vi "INI_bk5492c.vi"(5 "MCListbox Ref":refnum<vi>, 9 "MListBox Row":u16=2 max=8, 11 "Device INI Config File Path":path=path "D:/LABVIEW/SEQUENSER SNA/Ver 07/INI/DeviceConfig.ini") -> (0 "error out":errorcluster, 3 "Serial_VISA":T1)   [LabVIEW 2018]
uses:
  Examples - 32bit/SEQUENCER/SEQUENSER v10/Sequencer v10/Ctl/Serial_VISA.ctl
  <vilib>/Utility/miscctls.llb/LVRowAndColumnTypeDef.ctl
  <vilib>/Utility/config.llb/Read Key (String).vi
  <vilib>/Utility/config.llb/NI_LVConfig.lvlib
  <instrlib>/BK Precision 5490C Series/BK Precision 5490C Series.lvlib
panel:
  out "Array DMM":string[](array[string])
  out "DMM Read Buffer":string
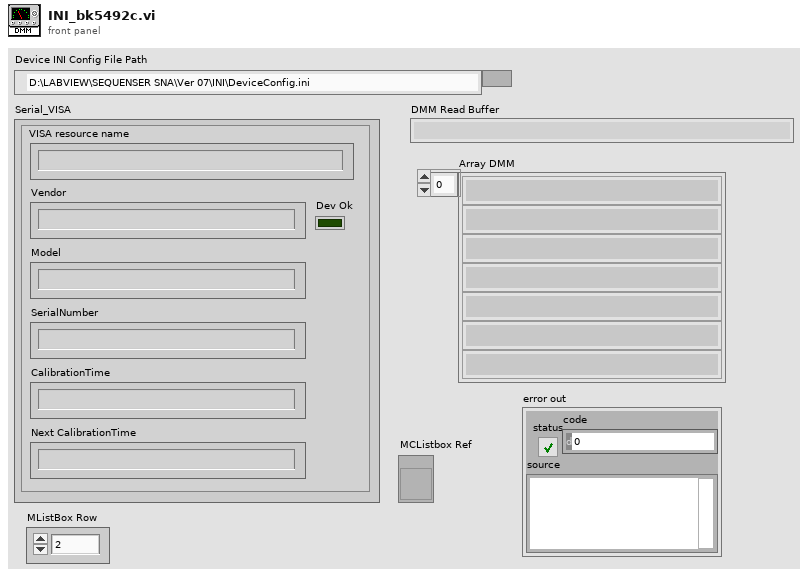
[diagram p1: front panel]
types:
  T1 = typedef "Serial_VISA.ctl" = cluster{"VISA resource name":string, "Vendor":string, "SerialNumber":string, "CalibrationTime":string, "Dev Ok":bool, "Model":string, "Next CalibrationTime":string}
  T2 = typedef "LVRowAndColumnTypeDef.ctl" = cluster{"Row":i32, "Column":i32}
  T3 = typedef "NI_LVConfig.lvlib/Config Data RefNum.ctl" = refnum<k1>
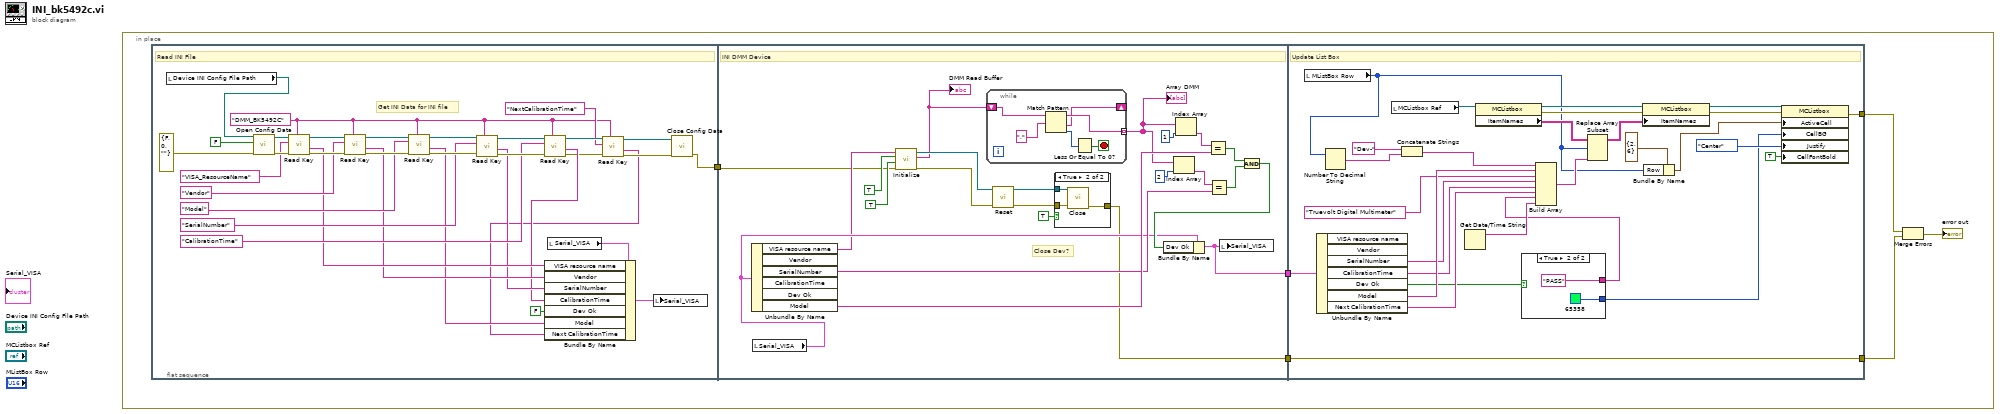
[diagram p0: block diagram]
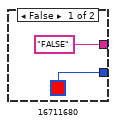
[diagram p3: hidden frame]
diagram:
  n1 = in-place {
    n2 = flat-sequence {
      tunnel: [w8] -> w6
      tunnel: w6 -> [w43]
      tunnel: [w49] -> w4
      tunnel: [w53] -> w1
      tunnel: [w81] -> w5
      tunnel: [w80] -> w3
      tunnel: w4 -> [w80]
      tunnel: w1 -> [w78]
      frame #0 {
        w13 = "DMM_BK5492C" ("section")
        # "Get INI Data for INI file"
        # "Read INI File"
        n3 = local read "Device INI Config File Path"() -> (w7:path)
        n4 = call <vilib>:"Open Config Data.vi"("error in (no error)"=errorcluster {"status"=FALSE, "code"=0, "source"=""} ("error constant"), "create file if necessary (T)"=FALSE, "configuration file path"=w7) -> ("error out"=w38:errorcluster, "refnum"=w39:T3)  [unwired: 6 in, 1 out]
        n5 = call-poly <vilib>:"Read Key.vi"("section"=w13, "error in (no error)"=w38, "key"="VISA_ResourceName", "refnum"=w39) -> ("error out"=w35:errorcluster, "value"=w24:string, "refnum out"=w37:T3)  [unwired: 4 in, 1 out]
        n6 = call-poly <vilib>:"Read Key.vi"("section"=w13, "error in (no error)"=w35, "key"="Vendor", "refnum"=w37) -> ("error out"=w34:errorcluster, "value"=w23:string, "refnum out"=w36:T3)  [unwired: 4 in, 1 out]
        n7 = call-poly <vilib>:"Read Key.vi"("section"=w13, "error in (no error)"=w34, "key"="Model", "refnum"=w36) -> ("error out"=w29:errorcluster, "value"=w22:string, "refnum out"=w30:T3)  [unwired: 4 in, 1 out]
        n8 = call-poly <vilib>:"Read Key.vi"("section"=w13, "error in (no error)"=w29, "key"="SerialNumber", "refnum"=w30) -> ("error out"=w26:errorcluster, "value"=w21:string, "refnum out"=w27:T3)  [unwired: 4 in, 1 out]
        n9 = call-poly <vilib>:"Read Key.vi"("section"=w13, "error in (no error)"=w26, "key"="CalibrationTime", "refnum"=w27) -> ("error out"=w17:errorcluster, "value"=w20:string, "refnum out"=w18:T3)  [unwired: 4 in, 1 out]
        n10 = local read "Serial_VISA"() -> (w10:T1)
        n11 = call-poly <vilib>:"Read Key.vi"("section"=w13, "error in (no error)"=w17, "key"="NextCalibrationTime", "refnum"=w18) -> ("error out"=w15:errorcluster, "value"=w12:string, "refnum out"=w16:T3)  [unwired: 4 in, 1 out]
        n12 = Bundle By Name(cluster=w10, "VISA resource name"=w24, "Vendor"=w23, "SerialNumber"=w21, "CalibrationTime"=w20, "Dev Ok"=FALSE, "Model"=w22, "Next CalibrationTime"=w12) -> (w9:T1)
        n13 = local write "Serial_VISA"(w9) -> ()
        n14 = call <vilib>:"Close Config Data.vi"("error in (no error)"=w15, "refnum"=w16) -> ("error out"=w8:errorcluster)  [unwired: 8 in, 1 out]
      }
      frame #1 {
        # "Close Dev?"
        # "INI DMM Device"
        n15 = local read "Serial_VISA"() -> (w54:T1)
        n16 = Unbundle By Name(w54) -> ("VISA resource name"=w48:string, "SerialNumber"=w58:string, "Model"=w61:string)  [unwired: 3 out]
        n17 = call <instrlib>:"Initialize.vi"("error in (no error)"=w43, "Reset (True)"=TRUE, "ID Query (True)"=TRUE, "VISA resource name"=w48) -> ("error out"=w44:errorcluster, "str parametrs"=w42:string, "VISA resource name out"=w47:refnum<visa-resource-name>)  [unwired: 5 in]
        "DMM Read Buffer" <- w42
        n18 = while {
          shift-right: [w70] -> _
          shift-left: w42 -> [w73]
          tunnel: [w71] -> w50 mode=indexing
          stop <- w68 stop-if-true
          n19 = Match Pattern(string=w73, regular expression="," ("search string/char (-)")) -> (before substring=w71:string, after substring=w70:string, offset past match=w69:i32)  [unwired: 1 in, 1 out]
          n20 = Less Or Equal To 0?(x=w69) -> (x <= 0?=w68:bool)
        }
        "Array DMM" <- w50
        n21 = call <instrlib>:"Reset.vi"("error in (no error)"=w44, "VISA resource name"=w47) -> ("error out"=w45:errorcluster, "VISA resource name out"=w46:refnum<visa-resource-name>)  [unwired: 8 in]
        n22 = case shown="True" TRUE {
          tunnel: [w64 w67] -> w49
          tunnel: w46 -> [_ w66]
          tunnel: w45 -> [w64 w65]
          frame False {
          }
          frame True {
            n23 = call <instrlib>:"Close.vi"("error in (no error)"=w65, "VISA resource name"=w66) -> ("error out"=w67:errorcluster)  [unwired: 9 in]
          }
        }
        n24 = Index Array(array=w50, index=2) -> (element=w60:string)
        n25 = Index Array(array=w50, index=1) -> (element=w62:string)
        n26 = Equal?(x=w62, y=w61) -> (x = y?=w57:bool)
        n27 = Equal?(x=w60, y=w58) -> (x = y?=w56:bool)
        n28 = And(x=w57, y=w56) -> (x .and. y?=w55:bool)
        n29 = Bundle By Name(cluster=w54, "Dev Ok"=w55) -> (w53:T1)
        n30 = local write "Serial_VISA"(w53) -> ()
      }
      frame #2 {
        # "Update List Box"
        n31 = local read "MListBox Row"() -> (w75:u16)
        n32 = Unbundle By Name(w78) -> ("SerialNumber"=w98:string, "CalibrationTime"=w99:string, "Dev Ok"=w84:bool, "Model"=w100:string, "Next CalibrationTime"=w101:string)  [unwired: 2 out]
        n33 = Number To Decimal String(number=w75) -> (decimal integer string=w77:string)  [unwired: 1 in]
        n34 = local read "MCListbox Ref"() -> (w88:refnum<vi>)
        n35 = Concatenate Strings("Dev-", w77) -> (w74:string)
        n36 = Get Date/Time String() -> (date string=w87:string)  [unwired: 3 in, 1 out]
        n37 = property class="MCListbox"(reference=w88) -> (reference out=w91:refnum<vi>, error out=w92:errorcluster, "ItemNames"=w93:string[][])  [unwired: 1 in]
        n38 = case shown="True" w84 {
          tunnel: [u32 16711680 u32 65358] -> w83
          tunnel: ["FALSE" ("element") "PASS" ("element")] -> w82
          frame False {
          }
          frame True {
          }
        }
        n39 = Build Array(w74, w100, "Truevolt Digital Multimeter", w98, w99, w101, w82, w87) -> (w95:string[])
        n40 = Replace Array Subset(array=w93, new element=w95, index (row)=w75) -> (w94:string[][])  [unwired: 1 in]
        n41 = property class="MCListbox"(reference=w91, error in=w92, "ItemNames"=w94) -> (reference out=w96:refnum<vi>, error out=w97:errorcluster)
        n42 = Bundle By Name(cluster=T2 {"Row"=2, "Column"=6} ("Active Cell:Active Cell"), "Row"=w75) -> (w85:T2)
        n43 = property class="MCListbox"(reference=w96, error in=w97, "ActiveCell"=w85, "CellBG"=w83, "Justify"=enum16{"Left", "Center", "Right"}."Center" ("Active Cell:Cell Justification"), "CellFontBold"=TRUE ("Active Cell:Cell Font:Bold")) -> (error out=w81:errorcluster)  [unwired: 1 out]
      }
    }
    n44 = Merge Errors(w5, w3) -> (→"error out":errorcluster)
  }
